vi "z view keyexpr from str unchecked.vi"(8 "error in (no error)":errorcluster, 10 "s":string, 11 "this_":cluster{}) -> (0 "error out":errorcluster, 3 "this_ out":cluster{})   [LabVIEW 2021, in "zenohc.lvlib"]
doc: "void z_view_keyexpr_from_str_unchecked(struct z_view_keyexpr_t *this_,\n const char *s);"
uses:
  zenohc.lvlib
  zenohc.dll
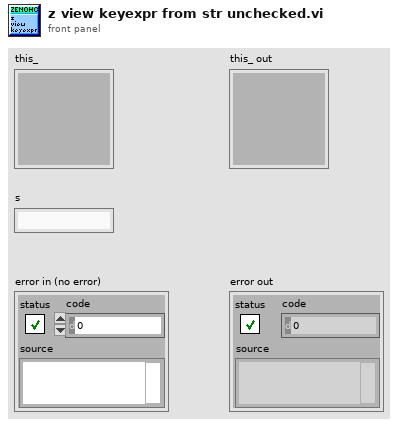
[diagram p1: front panel]
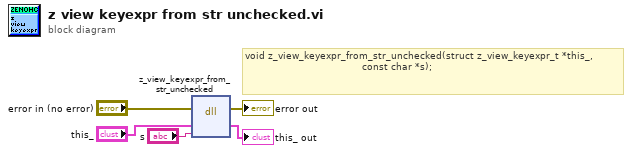
[diagram p0: block diagram]
diagram:
  # "void z_view_keyexpr_from_str_unchecked(struct z_view_keyexpr_t *this_,\n                                       const char *s);"
  n1 = dll-call lib="D:/dev/zenoh_labview/zenohc/zenohc.*" fn="z_view_keyexpr_from_str_unchecked"(error in="error in (no error)", "this_"="this_", "s"="s") -> (error out=→"error out":errorcluster, "this_"=→"this_ out":cluster{})  [unwired: 4 in, 1 out]
